vi "PV ActiveLine - SensorControl.vi"(0 "Referenz in":refnum<visa-resource-name>, 1 "controlling source activation":i32(ring)=2 items=["manual", "hotstart", "external", "by channel 1", "by channel 2"], 2 "controlling source deactivation":i32(ring)=2 items=["manual", "self", "external", "by channel 1", "by channel 2"], 3 "ON threshold":dbl=0.001 min=0.0 max=41000.0 format="%.2e", 4 "OFF threshold":dbl=0.001 min=0.0 max=41000.0 format="%.2e", 5 "Fehler (Eingang)":errorcluster, 6 "Gauge Nr.":i32(ring) items=["CH 1", "CH 2"], 8 "W/R":bool) -> (14 "Referenz out":refnum<visa-resource-name>, 15 "controlling source activation, out":i32(ring)=2 items=["manual", "hotstart", "external", "by channel 1", "by channel 2"], 16 "controlling source deactivation out":i32(ring)=2 items=["manual", "self", "external", "by channel 1", "by channel 2"], 17 "Get ON threshold":dbl min=0.0 max=41000.0 format="%.2e", 18 "Get OFF threshold":dbl min=0.0 max=41000.0 format="%.2e", 19 "Cluster (Ausgang)":errorcluster)   [LabVIEW 2013, in "PV ActiveLine.lvlib"]
doc: "SCx - Gauge Control\n\nTransmit: SCx [,a,b,c.ccEscc,d.ddEsdd]\n\nControlled gauge,\nx =\n1 –> Gauge 1\n2 –> Gauge 2\n\nGauge activation,\na =\n0 –> Manual (default)\n1 –> Hot start\n2 –> Via measurement channel 1\n3 –> Via measurement channel 2\n\nGauge deactivation,\nb =\n0 –> Manual (default)\n1 –> Self control\n2 –> Via measurement channel 1\n3 –> Via measurement channel 2\n\nON threshold\nOFF threshold"
uses:
  <instrlib>/PV ActiveLine/PV ActiveLine.lvlib
panel:
  # "mbar"
  # "mbar"
  # "mbar"
  # "mbar"
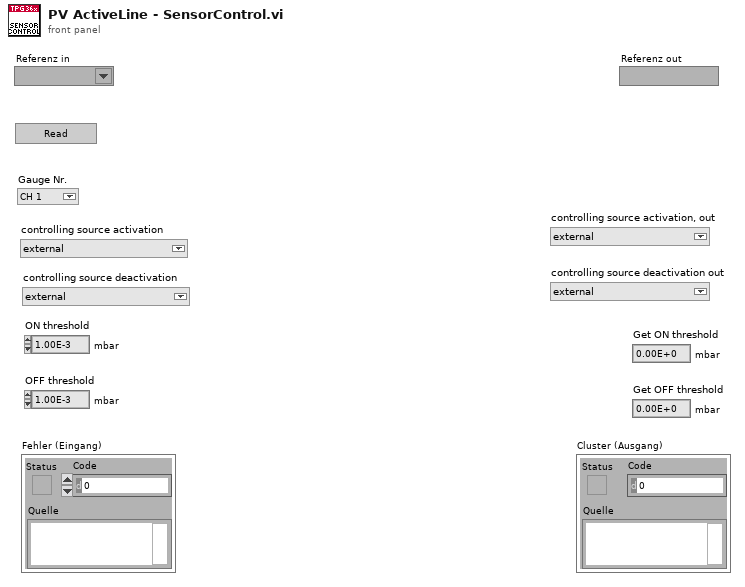
[diagram p1: front panel]
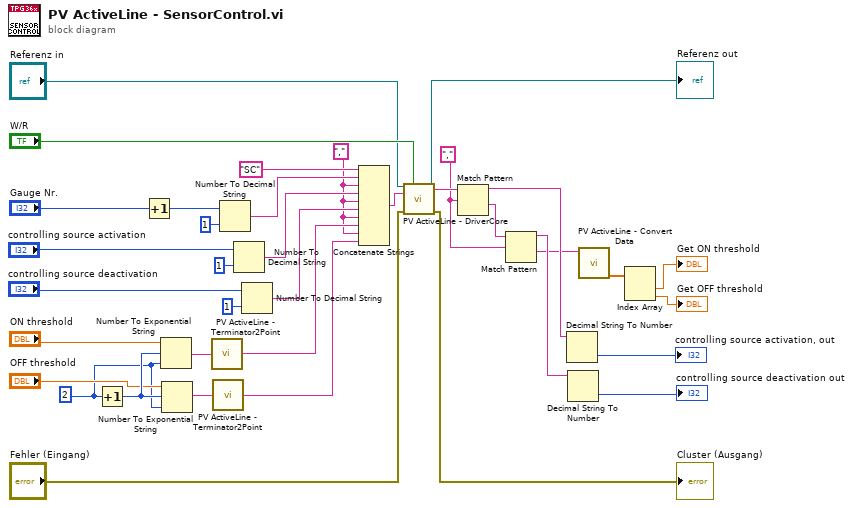
[diagram p0: block diagram]
diagram:
  w11 = 2
  w24 = "," ("Command")
  w10 = "," ("Command")
  n1 = Increment(x=w11) -> (x+1=w15:i32)
  n2 = Increment(x="Gauge Nr.") -> (x+1=w36:i32)
  n3 = Number To Exponential String(number="ON threshold", precision (6)=w11, 3:w15) -> (E-format string=w17:string)  [unwired: 1 in]
  n4 = Number To Exponential String(number="OFF threshold", precision (6)=w11, 3:w15) -> (E-format string=w16:string)  [unwired: 1 in]
  n5 = call <instrlib>:"PV ActiveLine - Terminator2Point.vi"("Eingangstring"=w17) -> ("Ausgangstring"=w14:string)
  n6 = call <instrlib>:"PV ActiveLine - Terminator2Point.vi"("Eingangstring"=w16) -> ("Ausgangstring"=w9:string)
  n7 = Number To Decimal String(number=w36, width (-)=i16 1) -> (decimal integer string=w31:string)
  n8 = Number To Decimal String(number="controlling source activation", width (-)=i16 1) -> (decimal integer string=w29:string)
  n9 = Number To Decimal String(number="controlling source deactivation", width (-)=i16 1) -> (decimal integer string=w28:string)
  n10 = Concatenate Strings("SC" ("Command"), w31, w10, w29, w10, w28, w10, w14, w10, w9) -> (w22:string)
  n11 = call <instrlib>:"PV ActiveLine - DriverCore.vi"("Referenz in"="Referenz in", "Write/Read"="W/R", "Command"=w22, "Fehler (Eingang)"="Fehler (Eingang)") -> ("Referenz out"=→"Referenz out":refnum<visa-resource-name>, "String Out"=w27:string, "Cluster (Ausgang)"=→"Cluster (Ausgang)":errorcluster)  [unwired: 9 in]
  n12 = Match Pattern(string=w27, regular expression=w24) -> (before substring=w26:string, after substring=w23:string)  [unwired: 1 in, 2 out]
  n13 = Match Pattern(string=w23, regular expression=w24) -> (before substring=w25:string, after substring=w8:string)  [unwired: 1 in, 2 out]
  n14 = Decimal String To Number(string=w26) -> (number=→"controlling source activation, out":i32)  [unwired: 2 in, 1 out]
  n15 = Decimal String To Number(string=w25) -> (number=→"controlling source deactivation out":i32)  [unwired: 2 in, 1 out]
  n16 = call <instrlib>:"PV ActiveLine - Convert Data.vi"("String in"=w8) -> ("DBL out"=w7:dbl[])  [unwired: 7 in, 3 out]
  n17 = Index Array(array=w7) -> (element #1=→"Get ON threshold":dbl, element #2=→"Get OFF threshold":dbl)  [unwired: 2 in]
